vi "GE 5565PIORC.DMA.Create Transfer.vi"   [LabVIEW 2017, in "GE 5565PIORC.lvclass"]
doc: "Creates a <B>DMA Transfer Spec</B> which associates a series of <B>Block Descriptors</B> to an offset in Reflective Memory."
uses:
  GE 5565PIORC.lvclass
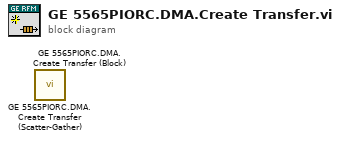
[diagram p0: block diagram]
diagram:
  n1 = call "GE 5565PIORC.DMA.Create Transfer (Scatter-Gather).vi"() -> ()  [unwired: 8 in, 4 out]
  n2 = call "GE 5565PIORC.DMA.Create Transfer (Block).vi"() -> ()  [unwired: 8 in, 4 out]
